vi "Ouptut_Sound_trace_ph2.vi"() -> (5 "Plug in titles":string[](array[string]), 7 "Plug in values":string[](array[string]))   [LabVIEW 2011]
doc: "This VI demonstrates how to output continuous sound using SO Set Num Buffers. This example is available only on Windows."
uses:
  <vilib>/sound2/lvsound2.llb/Sound Data Format.ctl
  <vilib>/sound2/lvsound2.llb/Sampling Mode.ctl
  Globals/Meas_global.vi
  <vilib>/sound2/lvsound2.llb/Sound Output Write (DBL Single).vi
  <vilib>/measure/NI_MABase.lvlib
panel:
  in  "Dwell Time (s)":dbl=0.1
  in  "Desired Amplitudes":dbl[](array[numeric])=[0.1, 0.15, 0.25]
  in  "Desired Frequencies":dbl[](array[numeric])=[1000.0, 2000.0, 2500.0, 3500.0]
  in  "Number of Cycles":i32=100
  out "Generated Sound":waveform(dbl)(graph)={"t0"=timestamp(0 s since 1904-01-01), "dt"=2.2675736961451248e-05, "Y"=[]}
  out "Loop count":i32=4
  in  "Device ID":u32
  in  "Sound Format":T1={"sample rate (S/s)"=44100.0, "number of channels"=1, "bits per sample"=16}
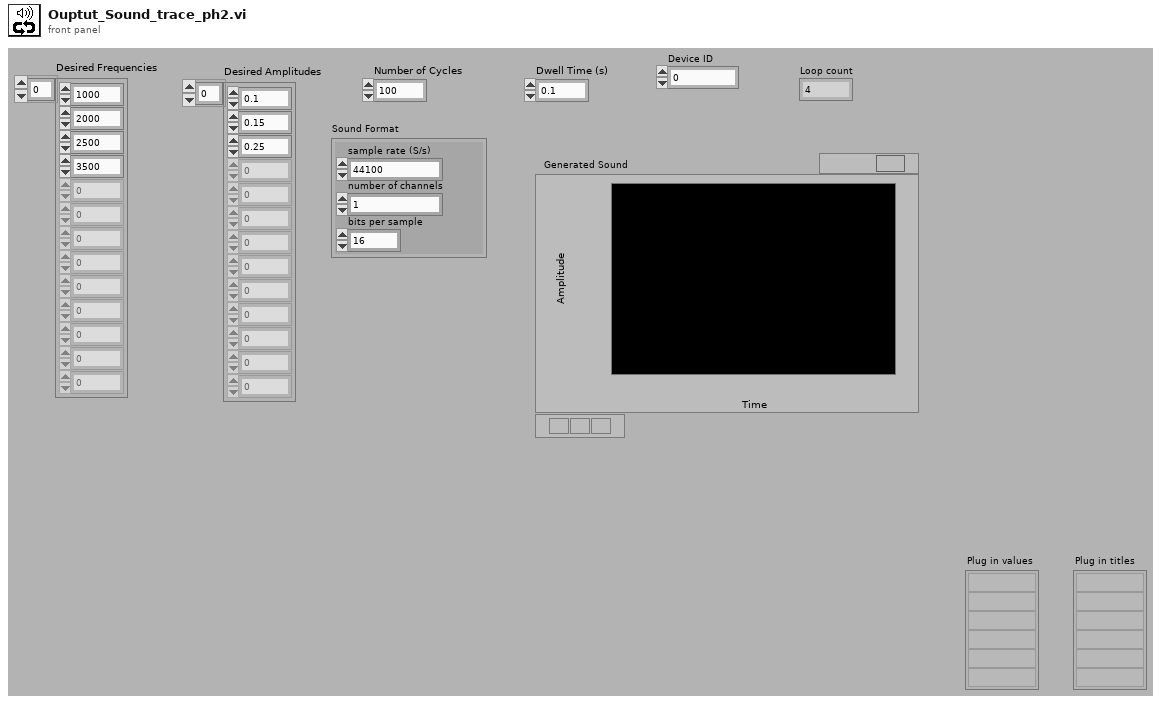
[diagram p1: front panel]
types:
  T1 = typedef "Sound Data Format.ctl" = cluster{"sample rate (S/s)":dbl, "number of channels":i32, "bits per sample":i32}
  T2 = typedef "Post_Process.ctl" = enum16{"Take New Data", "Post Process Raw Data File"}
  T3 = typedef "Sampling Mode.ctl" = i32
  T4 = typedef "Sound Output Task ID.ctl" = u32
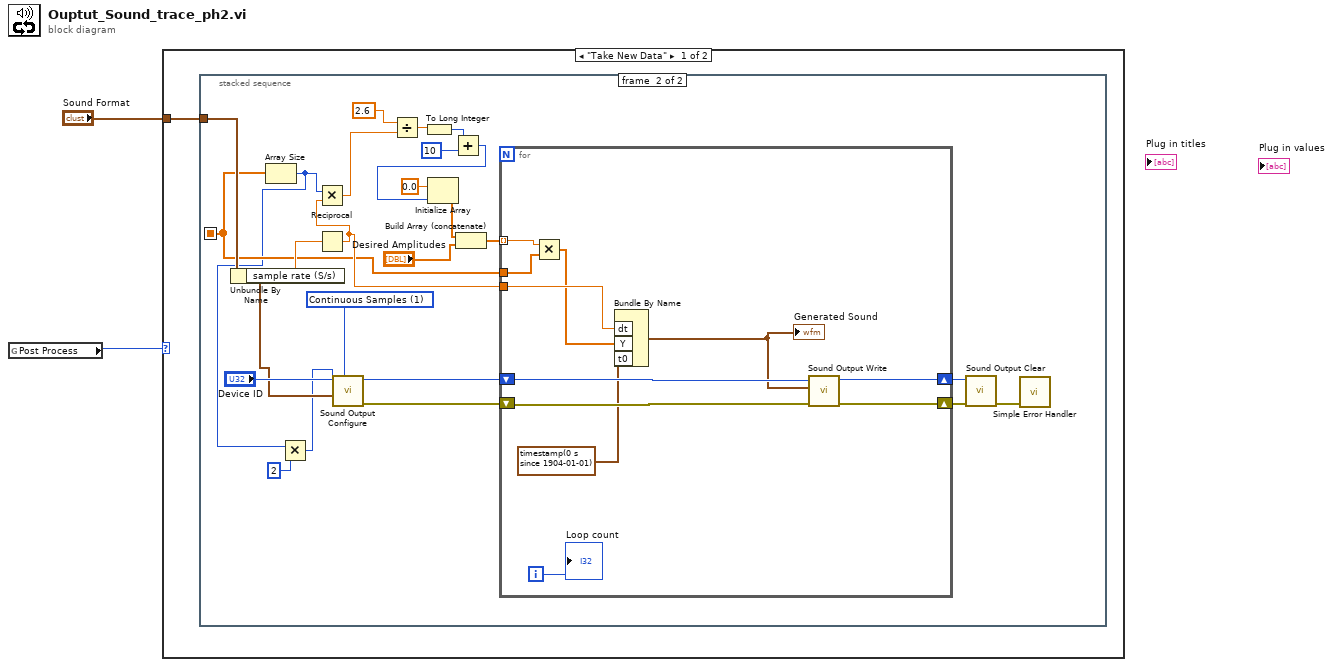
[diagram p0: block diagram]
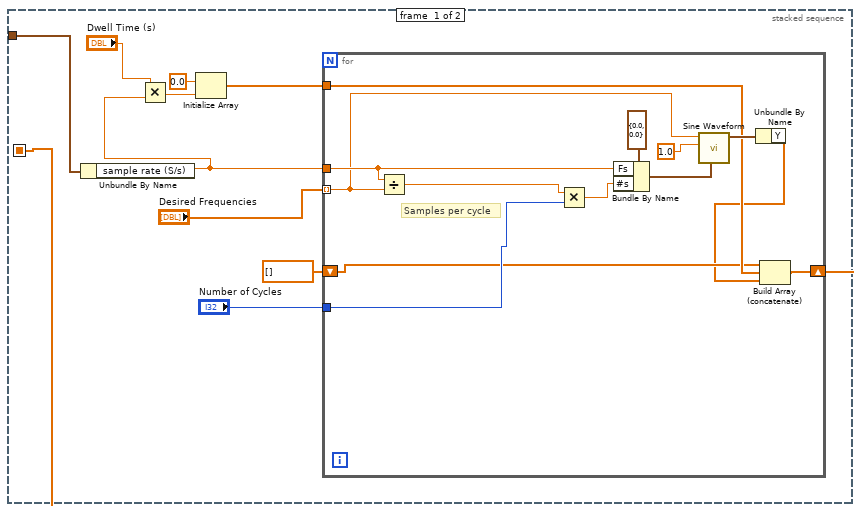
[diagram p2: hidden frame]
diagram:
  n1 = global read "Meas_global.vi" "Post Process"() -> (w2:T2)
  n2 = case shown="\"Take New Data\"" w2 {
    tunnel: "Sound Format" -> [w3 _]
    frame "Take New Data" {
      n3 = stacked-sequence {
        seq-local: [w4 _] -> [_ w33]
        tunnel: w3 -> [w13 w43]
        frame #0 {
          n4 = Unbundle By Name(w13) -> ("sample rate (S/s)"=w10:dbl)
          n5 = Multiply(x="Dwell Time (s)", y=w10) -> (x*y=w8:dbl)
          n6 = Initialize Array(0.0 ("element"), w8) -> (w6:dbl[])
          n7 = for {
            tunnel: w10 -> [w25]
            tunnel: "Desired Frequencies" -> [w15] mode=indexing
            tunnel: "Number of Cycles" -> [w24]
            shift-right: [w16] -> w4
            shift-left: dbl[] [] -> [w17]
            tunnel: w6 -> [w18]
            # "Samples per cycle"
            n8 = Divide(x=w25, y=w15) -> (x/y=w21:dbl)
            n9 = Multiply(x=w21, y=w24) -> (x*y=w23:dbl)
            n10 = Bundle By Name(cluster=cluster{"Fs":dbl, "#s":dbl} {"Fs"=0.0, "#s"=0.0} ("sampling info"), "Fs"=w25, "#s"=w23) -> (w20:cluster{"Fs":dbl, "#s":dbl})
            n11 = call <vilib>:"Sine Waveform.vi"("sampling info"=w20, "amplitude"=1.0, "frequency"=w15) -> ("signal out"=w19:waveform(dbl))  [unwired: 7 in, 1 out]
            n12 = Unbundle By Name(w19) -> ("Y"=w14:dbl[])
            n13 = Build Array (concatenate)(w17, w18, w14) -> (w16:dbl[])
          }
        }
        frame #1 {
          w45 = T3 1 items=["Finite Samples", "Continuous Samples"] ("sample mode")
          n14 = Unbundle By Name(w43) -> ("sample rate (S/s)"=w42:dbl)
          n15 = Array Size(array=w33) -> (size(s)=w27:i32)
          n16 = Multiply(x=w27, y=2) -> (x*y=w28:i32)
          n17 = Reciprocal(x=w42) -> (1/x=w35:dbl)
          n18 = Multiply(x=w27, y=w35) -> (x*y=w40:dbl)
          n19 = call <vilib>:"Sound Output Configure.vi"("number of samples/ch"=w28, "sample mode"=w45, "sound format"=w43, "device ID"="Device ID") -> ("error out"=w50:errorcluster, "task ID"=w49:T4)  [unwired: 6 in]
          n20 = Divide(x=2.6, y=w40) -> (x/y=w39:dbl)
          n21 = To Long Integer(number=w39) -> (32bit integer=w32:i32)
          n22 = Add(x=w32, y=10) -> (x+y=w31:i32)
          n23 = Initialize Array(0.0 ("element"), w31) -> (w36:dbl[])
          n24 = Build Array (concatenate)(w36, "Desired Amplitudes") -> (w34:dbl[])
          n25 = for {
            shift-right: [w57] -> w48
            shift-left: w50 -> [w59]
            shift-right: [w61] -> w47
            shift-left: w49 -> [w58]
            tunnel: w35 -> [w55]
            tunnel: w34 -> [w53] mode=indexing
            tunnel: w33 -> [w52]
            i -> [w60]
            n26 = Multiply(x=w53, y=w52) -> (x*y=w54:dbl[])
            n27 = Bundle By Name("dt"=w55, "Y"=w54, "t0"=timestamp(0 s since 1904-01-01)) -> (w51:waveform(dbl))  [unwired: 1 out]
            "Generated Sound" <- w51
            n28 = call-poly <vilib>:"Sound Output Write.vi"("error in (no error)"=w59, "data"=w51, "task ID"=w58) -> ("error out"=w57:errorcluster, "task ID out"=w61:T4)  [unwired: 7 in]
            "Loop count" <- w60
          }
          n29 = call <vilib>:"Sound Output Clear.vi"("error in (no error)"=w48, "task ID"=w47) -> ("error out"=w44:errorcluster)  [unwired: 9 in]
          n30 = call <vilib>:"Simple Error Handler.vi"("error in (no error)"=w44) -> ()  [unwired: 4 in, 5 out]
        }
      }
    }
    frame "Post Process Raw Data File" {
    }
  }
